vi "LinCheck Protokoll FT-IR.vi"(0 "Eingabetabelle":T17, 5 "Sprachliste":string[][](array[string]), 7 "Lin-Polynom Daten":T1 {"zusätzliche Zeitdauer Erster Punkt" format="%#_5g"; "Lin Modus" items=["Cal Gas to PNS", "Cal Gas to Samplepoint", "Measure"]; "Gas Ablaufdatum" format="%<%d.%m.%Y>T"; "HovaCAL Flow AutoLin"."HovaCAL Flow Input Cluster" format="%.2f"; "Gasflasche" items=["----"=10000, "IAG MG"=0, "IAG NH3 3000"=1, "IAG NH3 2000"=2, "IAG NH3 200"=3]; "Conditions:" items=["field", "laboratory"]; "Kalibrierauswahl" items=["Inaktiv", "Aktiv"]; "Anzahl Stufen" format="%#_5g"; "Zeitdauer Stufe" format="%#_5g"; "Verdünnungsgas" items=["N2", "O2"]; "Komponentenauswahl"."Konzentration" format="%#.6f"; "Gasnummer:" min=1 max=5; "Prüfgas Konzentration" format="%#.6f"; "Polynomkoeff." format="%#_18f"}, 11 "error in (no error)":errorcluster caption="Fehler (Eingang, kein Fehler)") -> (4 "Eingabetabelle erweitert":string[][](array[string]), 6 "Ergebnis":string[][](array[string]), 8 "Aktiv":T15, 10 "bestanden":bool, 14 "Lin-Polynom Daten":T1 {"zusätzliche Zeitdauer Erster Punkt" format="%#_5g"; "Lin Modus" items=["Cal Gas to PNS", "Cal Gas to Samplepoint", "Measure"]; "Gas Ablaufdatum" format="%<%d.%m.%Y>T"; "HovaCAL Flow AutoLin"."HovaCAL Flow Input Cluster" format="%.2f"; "Gasflasche" items=["----"=10000, "IAG MG"=0, "IAG NH3 3000"=1, "IAG NH3 2000"=2, "IAG NH3 200"=3]; "Conditions:" items=["field", "laboratory"]; "Kalibrierauswahl" items=["Inaktiv", "Aktiv"]; "Anzahl Stufen" format="%#_5g"; "Zeitdauer Stufe" format="%#_5g"; "Verdünnungsgas" items=["N2", "O2"]; "Komponentenauswahl"."Konzentration" format="%#.6f"; "Gasnummer:" min=1 max=5; "Prüfgas Konzentration" format="%#.6f"; "Polynomkoeff." format="%#_18f"}, 15 "error out":errorcluster caption="Fehler (Ausgang)")   [LabVIEW 2020, in "Linearisierung v2.lvlib"]
doc: "Bereitet die Messdaten und die Linearisierungs-Polynom-Daten zu zwei 2D-Arrays (String) auf,die direkt in einem Tabellenelement angezeigt oder in einer Textdatei gespeichert werden können."
uses:
  Linearisierung v2.lvlib
  Lin-Polynom Daten.ctl
  KomponentenArray.ctl
  Visualisierungs Elemente/Auswahlfeld.ctl
  Visualisierungs Elemente/Zahlen-Eingabefeld.ctl
  EPA Optionsfeld.ctl
  Gasteiler/HovaCal/AutoLin Hovacal.ctl
  Kalibrieroption.ctl
  EPA1065-307/Condition.ctl
  Seiten/System Einstellungen V2/Konfig Gasflasche.ctl
  Seiten/System Einstellungen V2/Gasflasche Auswahl.ctl
  Gasteiler/HovaCAL_Interface/Controls/Flow Einstellung.ctl
  Gasteiler/HovaCAL_Interface/Controls/Pump state.ctl
  Seiten/CalGas Aufschaltung/Lin Modus.ctl
  Eingabetabelle.ctl
  AktivArray.ctl
  AktivButton.ctl
  AutoLin Protokoll/AutoLin Protokoll.lvlib
  Allgemein/allgemeine Sub-VIs.lvlib
  SpanEinstellungen/SpanEinstellungen.lvlib
  Gasteiler/Gasteiler.lvlib
  Gasteiler/HovaCal/HovaCal.lvlib
  EPA1065-307/Linearity verification 1065-307.lvlib
  Seiten/System Einstellungen V2/System Einstellungen V2.lvlib
  Gasteiler/HovaCAL_Interface/Controls/Controls.lvlib
  Seiten/CalGas Aufschaltung/CalGas Aufschaltung.lvlib
panel:
  # "Gasteiler (ppm)"
  # "Messgerät (ppm)"
  # "%"
  # "%"
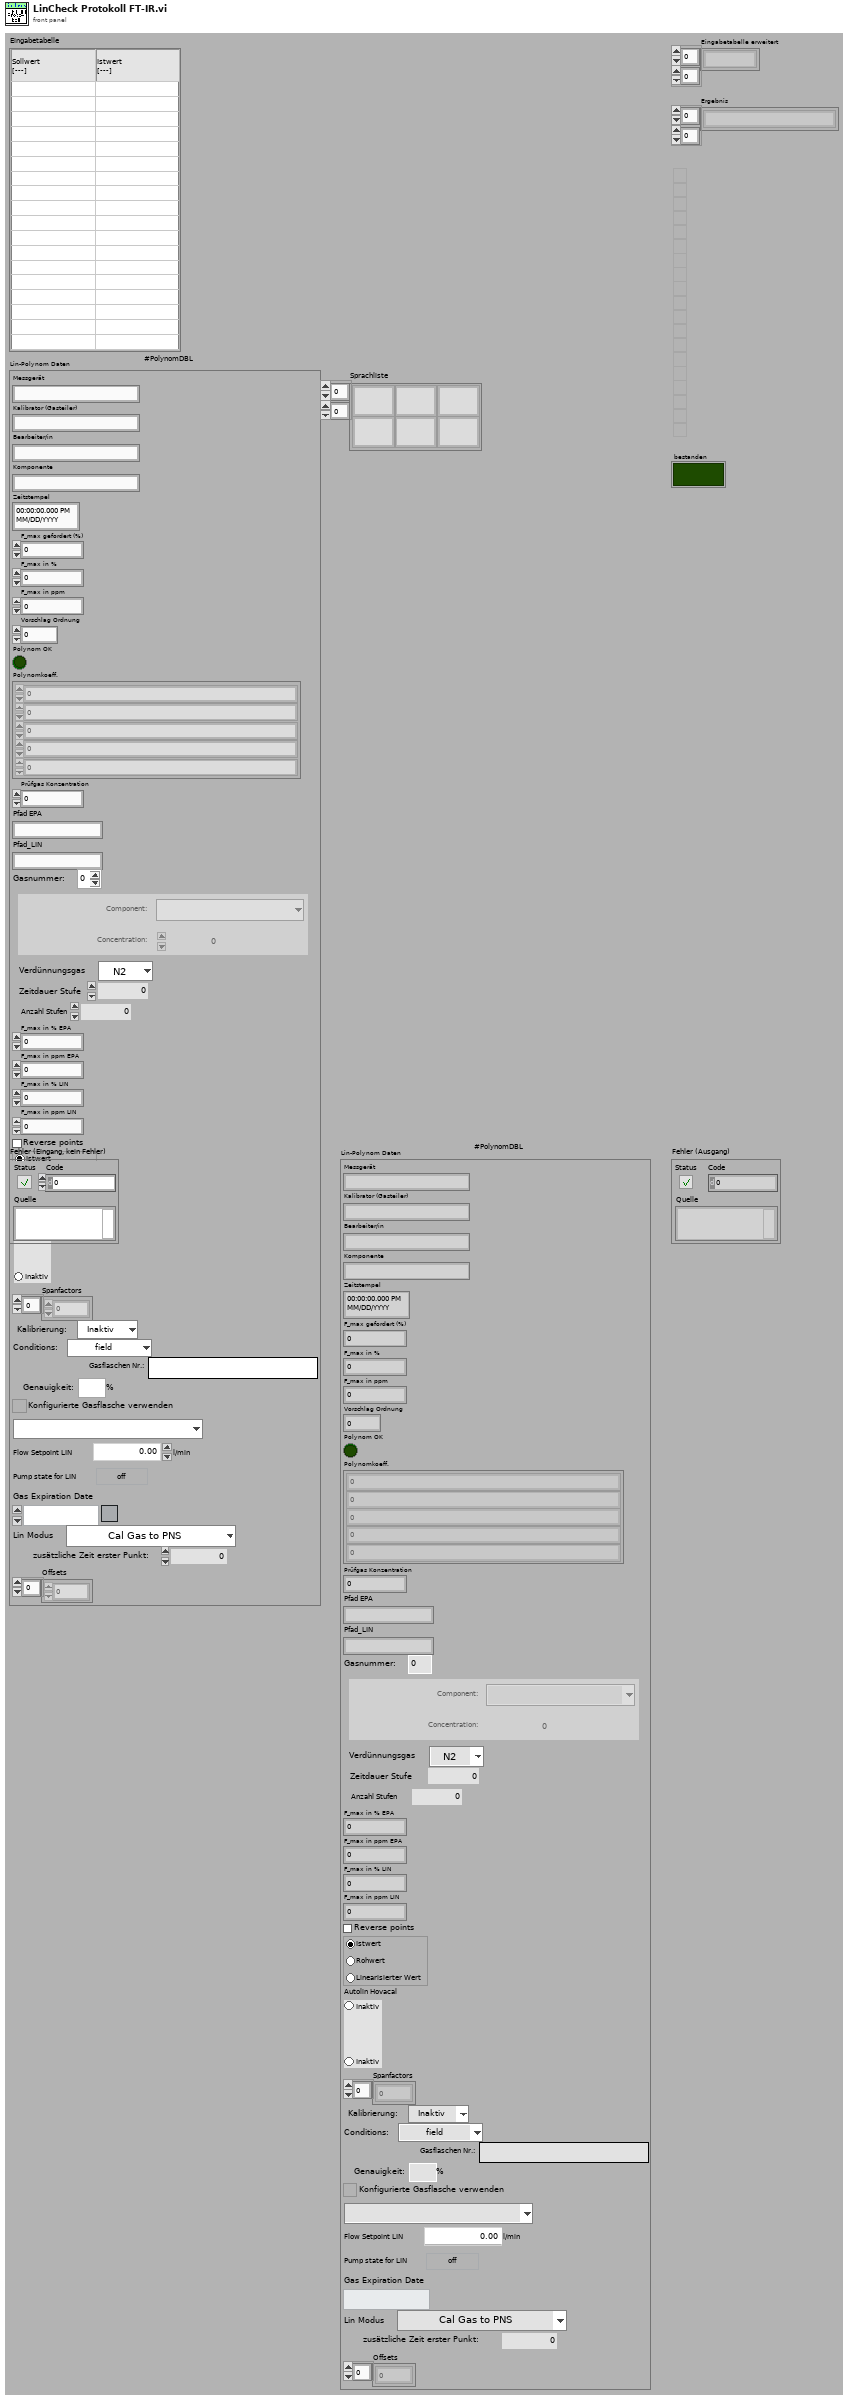
[diagram p1: front panel]
types:
  T1 = typedef "Linearisierung v2.lvlib/Lin-Polynom Daten.ctl" = cluster{"Messgerät":string, "Kalibrator (Gasteiler)":string, "Bearbeiter/in":string, "Komponente":string, "Zeitstempel":timestamp, "F_max gefordert (%)":sgl, "F_max in %":sgl, "F_max in ppm":sgl, "Vorschlag Ordnung":i32, "Polynom OK":bool, "Polynomkoeff.":dbl[], "Prüfgas Konzentration":dbl, "Pfad EPA":string, "Pfad_LIN":string, "Gasnummer:":u8, "Komponentenauswahl":T2, "Verdünnungsgas":T4, "Zeitdauer Stufe":T5, "Anzahl Stufen":T5, "F_max in % EPA":sgl, "F_max in ppm EPA":sgl, "F_max in % LIN":sgl, "F_max in ppm LIN":sgl, "Punkte umkehren":bool, "EPA Optionsfeld":T6, "Autolin Hovacal":T7, "Spanfactors":sgl[], "Kalibrierauswahl":T8, "Conditions:":T9, "Gasflaschen Nr.:":string, "Bottle Accuracy":dbl, "Konfig Gasflasche":T10, "Gasflasche":T11, "HovaCAL Flow AutoLin":T12, "MFC Output":T13, "Gas Ablaufdatum":timestamp, "Lin Modus":T14, "zusätzliche Zeitdauer Erster Punkt":sgl, "Offsets":sgl[]}
  T2 = typedef "Linearisierung v2.lvlib/KomponentenArray.ctl" = cluster{"Komponente:":T3, "Konzentration":dbl}[]
  T3 = typedef "Auswahlfeld.ctl" = u16
  T4 = typedef "Linearisierung v2.lvlib/Gasteiler.lvlib/Prüfgas in.ctl" = u16
  T5 = typedef "Zahlen-Eingabefeld.ctl" = sgl
  T6 = typedef "Linearisierung v2.lvlib/EPA Optionsfeld.ctl" = enum32{"Istwert", "Rohwert", "Linearisierter Wert"}
  T7 = typedef "Linearisierung v2.lvlib/Gasteiler.lvlib/HovaCal.lvlib/AutoLin Hovacal.ctl" = enum32{"Keine Auswahl", "Optionsauswahl 1", "Optionsauswahl 2"}
  T8 = typedef "Linearisierung v2.lvlib/Kalibrieroption.ctl" = u16
  T9 = typedef "Linearisierung v2.lvlib/Linearity verification 1065-307.lvlib/Condition.ctl" = u16
  T10 = typedef "System Einstellungen V2.lvlib/Konfig Gasflasche.ctl" = bool
  T11 = typedef "System Einstellungen V2.lvlib/Gasflasche Auswahl.ctl" = u16
  T12 = typedef "Linearisierung v2.lvlib/Gasteiler.lvlib/HovaCAL_Interface.lvlib/Controls.lvlib/Flow Einstellung.ctl" = cluster{"HovaCAL Flow Input Cluster":dbl}
  T13 = typedef "Linearisierung v2.lvlib/Gasteiler.lvlib/HovaCAL_Interface.lvlib/Controls.lvlib/Pump state.ctl" = cluster{"Run":bool}
  T14 = typedef "CalGas Aufschaltung.lvlib/Lin Modus.ctl" = u16
  T15 = typedef "Linearisierung v2.lvlib/AktivArray.ctl" = T16[]
  T16 = typedef "Linearisierung v2.lvlib/AktivButton.ctl" = bool
  T17 = typedef "Linearisierung v2.lvlib/Eingabetabelle.ctl" = string[][]
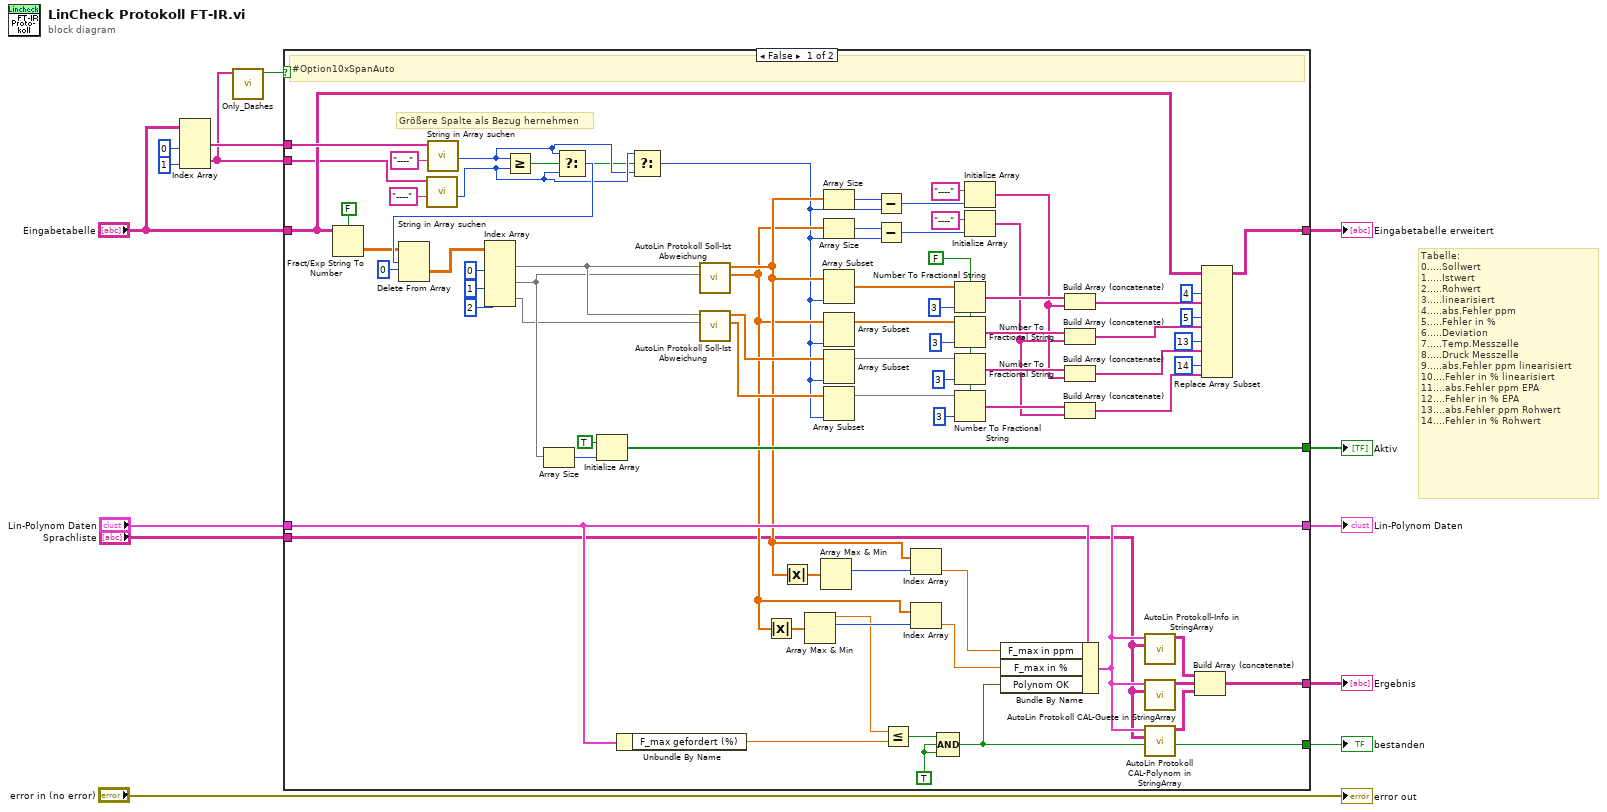
[diagram p0: block diagram]
diagram:
  # "Tabelle:\n0.....Sollwert\n1.....Istwert\n2.....Rohwert\n3.....linearisiert\n4.....abs.Fehler ppm\n5.....Fehler in %\n6.....Deviation\n7.....Temp.Messzelle\n8.....Druck Messzelle\n9.....abs.Fehler ppm linearisiert\n10....Fehler in % linearisiert\n11....abs.Fehler ppm EPA\n12....Fehler in % EPA\n13....abs.Fehler ppm Rohwert\n14....Fehler in % Rohwert"
  n1 = Index Array(array="Eingabetabelle", index (col) #1=0 ("Deaktivierter Index (Spalte)"), index (col) #2=1 ("Index (Spalte)")) -> (element #1=w8:string[], element #2=w3:string[])  [unwired: 2 in]
  n2 = call "Only_Dashes.vi"("Eingabetabelle"=w3) -> ("Dashes_only"=w2:bool)  [unwired: 10 in]
  n3 = case shown="False" w2 {
    tunnel: [w77 _] -> w14
    tunnel: [w76 _] -> w13
    tunnel: [w71 w91] -> w12
    tunnel: [w67 w90] -> w11
    tunnel: "Lin-Polynom Daten" -> [w66 w90]
    tunnel: [w51 _] -> w9
    tunnel: w8 -> [w47 _]
    tunnel: "Eingabetabelle" -> [w45 w91]
    tunnel: w3 -> [w38 _]
    tunnel: "Sprachliste" -> [w15 _]
    frame False {
      w40 = FALSE ("Systemdezimalzeichen verwenden (T)")
      w78 = TRUE ("Wert")
      # "Größere Spalte als Bezug hernehmen"
      # "#Option10xSpanAuto"
      n4 = Fract/Exp String To Number(use system decimal point (T)=FALSE ("Systemdezimalzeichen verwenden (T)"), string=w45) -> (number=w42:dbl[][])  [unwired: 2 in, 1 out]
      n5 = call "String in Array suchen.vi"("Nach String/Zeichen suchen (-)"="----", "String-Array"=w38) -> ("Index"=w37:i32)  [unwired: 7 in, 2 out]
      n6 = call "String in Array suchen.vi"("Nach String/Zeichen suchen (-)"="----", "String-Array"=w47) -> ("Index"=w36:i32)  [unwired: 7 in, 2 out]
      n7 = Greater Or Equal?(x=w36, y=w37) -> (x >= y?=w35:bool)
      n8 = Select(t=w36, s=w35, f=w37) -> (s? t:f=w43:i32)
      n9 = Delete From Array(array=w42, length=w43, index (row)=0 ("Index (Zeile)")) -> (deleted portion=w41:dbl[][])  [unwired: 1 in, 1 out]
      n10 = Index Array(array=w41, index (col) #1=0 ("Deaktivierter Index (Spalte)"), index (col) #2=1 ("Index (Spalte)"), index (col) #3=2 ("Index (Spalte)")) -> (element #1=w52:dbl[], element #2=w50:dbl[], element #3=w49:dbl[])  [unwired: 3 in]
      n11 = Array Size(array=w50) -> (size(s)=w64:i32)
      n12 = Initialize Array(TRUE, w64) -> (w51:bool[])
      n13 = Unbundle By Name(w66) -> ("F_max gefordert (%)"=w86:sgl)
      n14 = Select(t=w37, s=w35, f=w36) -> (s? t:f=w26:i32)
      n15 = call "AutoLin Protokoll Soll-Ist Abweichung.vi"("Istwerte (ppm)"=w50, "Sollwerte (ppm)"=w52) -> ("% vom Sollwert"=w29:sgl[], "abs. Fehler (ppm)"=w33:sgl[])  [unwired: 7 in, 1 out]
      n16 = call "AutoLin Protokoll Soll-Ist Abweichung.vi"("Istwerte (ppm)"=w49, "Sollwerte (ppm)"=w52) -> ("% vom Sollwert"=w57:sgl[], "abs. Fehler (ppm)"=w58:sgl[])  [unwired: 7 in, 1 out]
      n17 = Absolute Value(x=w29) -> (abs(x)=w84:sgl[])
      n18 = Absolute Value(x=w33) -> (abs(x)=w85:sgl[])
      n19 = Array Max & Min(array=w84) -> (max value=w65:sgl, max index (indices)=w80:i32)  [unwired: 2 out]
      n20 = Array Max & Min(array=w85) -> (max index (indices)=w82:i32)  [unwired: 3 out]
      n21 = Array Size(array=w33) -> (size(s)=w32:i32)
      n22 = Array Size(array=w29) -> (size(s)=w30:i32)
      n23 = Array Subset(array=w33, length=w26) -> (w34:sgl[])  [unwired: 1 in]
      n24 = Array Subset(array=w29, length=w26) -> (w31:sgl[])  [unwired: 1 in]
      n25 = Array Subset(array=w58, length=w26) -> (w28:sgl[])  [unwired: 1 in]
      n26 = Array Subset(array=w57, length=w26) -> (w27:sgl[])  [unwired: 1 in]
      n27 = Subtract(x=w32, y=w26) -> (x-y=w24:i32)
      n28 = Subtract(x=w30, y=w26) -> (x-y=w22:i32)
      n29 = Less Or Equal?(x=w65, y=w86) -> (x <= y?=w79:bool)
      n30 = Index Array(array=w33, index=w82) -> (element=w83:sgl)
      n31 = Index Array(array=w29, index=w80) -> (element=w81:sgl)
      n32 = Compound Arithmetic op=AND(w79, w78, w78) -> (w77:bool)
      n33 = Number To Fractional String(use system decimal point (T)=w40, number=w34, precision (6)=i16 3 ("Genauigkeit (6)")) -> (F-format string=w75:string[])  [unwired: 1 in]
      n34 = Number To Fractional String(use system decimal point (T)=w40, number=w31, precision (6)=i16 3 ("Genauigkeit (6)")) -> (F-format string=w72:string[])  [unwired: 1 in]
      n35 = Number To Fractional String(use system decimal point (T)=w40, number=w28, precision (6)=i16 3 ("Genauigkeit (6)")) -> (F-format string=w56:string[])  [unwired: 1 in]
      n36 = Number To Fractional String(use system decimal point (T)=w40, number=w27, precision (6)=i16 3 ("Genauigkeit (6)")) -> (F-format string=w55:string[])  [unwired: 1 in]
      n37 = Initialize Array("----" ("Nach String/Zeichen suchen (-)"), w24) -> (w18:string[])
      n38 = Initialize Array("----" ("Nach String/Zeichen suchen (-)"), w22) -> (w16:string[])
      n39 = Bundle By Name(cluster=w66, "F_max in ppm"=w83, "F_max in %"=w81, "Polynom OK"=w77) -> (w67:T1)
      n40 = Build Array (concatenate)(w75, w18) -> (w21:string[])
      n41 = Build Array (concatenate)(w72, w16) -> (w20:string[])
      n42 = Build Array (concatenate)(w56, w18) -> (w19:string[])
      n43 = Build Array (concatenate)(w55, w16) -> (w17:string[])
      n44 = call "AutoLin Protokoll-Info in StringArray.vi"("Sprachliste"=w15, "Lin-Polynom"=w67) -> ("Protokoll-Info-String"=w70:string[][])  [unwired: 9 in]
      n45 = call "AutoLin Protokoll CAL-Guete in StringArray.vi"("Sprachliste"=w15, "Lin-Polynom"=w67) -> ("Lin-Güte (Protokoll)"=w69:string[][])  [unwired: 9 in]
      n46 = call "AutoLin Protokoll CAL-Polynom in StringArray.vi"("Sprachliste"=w15, "Lin-Polynom"=w67) -> ("LinPolynom (Protokoll)"=w68:string[][])  [unwired: 9 in]
      n47 = Build Array (concatenate)(w70, w69, w68) -> (w76:string[][])
      n48 = Replace Array Subset(array=w45, new element #1=w21, index (col) #1=4 ("Deaktivierter Index (Spalte)"), new element #2=w20, index (col) #2=5 ("Index (Spalte)"), new element #3=w19, index (col) #3=13 ("Index (Spalte)"), new element #4=w17, index (col) #4=14 ("Index (Spalte)")) -> (w71:T17)  [unwired: 4 in]
    }
    frame True {
    }
  }
  "Eingabetabelle erweitert" <- w12
  "Ergebnis" <- w13
  "bestanden" <- w14
  "Aktiv" <- w9
  "Lin-Polynom Daten" <- w11
  "error out" <- "error in (no error)"
